vi "Post (Variant).vi"(6 "timestamp in":timestamp, 7 "PV name":string, 8 "error in (no error)":errorcluster, 10 "value in":variant, 11 "Server in":refnum<class "Server.lvclass">) -> (0 "error out":errorcluster, 2 "value out":variant, 3 "Server out":refnum<class "Server.lvclass">, 4 "timestamp out":timestamp)   [LabVIEW 2020, in "PV Access.lvlib" / "PVA Server.lvlib" / "Server.lvclass"]
uses:
  Server.lvclass
  Server.lvclass/Server.ctl
  f8dd957a-a825-461c-8340-a5d995baafef.vi
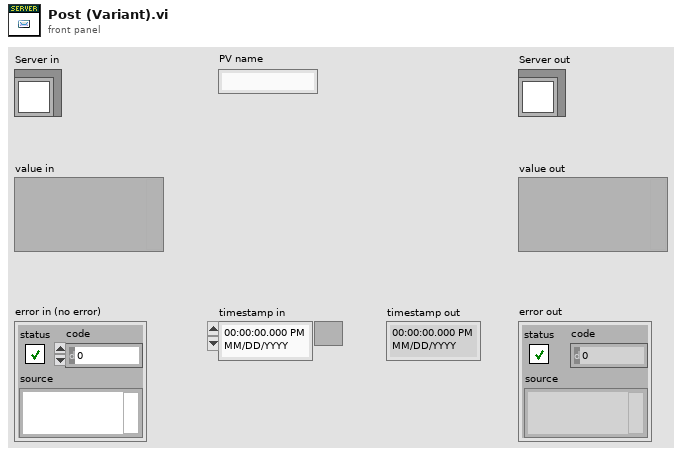
[diagram p1: front panel]
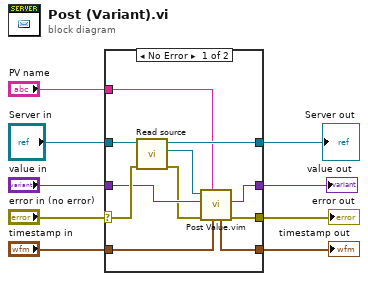
[diagram p0: block diagram]
diagram:
  n1 = case shown="No Error" "error in (no error)" {
    selector: "error in (no error)" -> [w16 w24]
    tunnel: [w17 w24] -> w3
    tunnel: [w19 w23] -> w1
    tunnel: "Server in" -> [w20 w23]
    tunnel: "PV name" -> [w10 _]
    tunnel: "value in" -> [w12 w22]
    tunnel: [w18 w22] -> w4
    tunnel: "timestamp in" -> [w15 w21]
    tunnel: [w14 w21] -> w2
    frame No Error {
      n2 = call "Read source.vi"("error in (no error)"=w16, "Server in"=w20) -> ("error out"=w11:errorcluster, "Source"=w13:refnum<class "Source.lvclass">, "Server out"=w19:refnum<class "Server.lvclass">)  [unwired: 7 in]
      n3 = call "Post Value.vim"("timestamp in"=w15, "PV name"=w10, "error in"=w11, "value in"=w12, "Source in"=w13) -> ("error out"=w17:errorcluster, "value out"=w18:variant, "timestamp out"=w14:timestamp)  [unwired: 3 in, 1 out]
    }
    frame Error {
    }
  }
  "error out" <- w3
  "Server out" <- w1
  "value out" <- w4
  "timestamp out" <- w2
